vi "Basic Averaged DC-RMS for 1 Chan.vi"(7 "reset":bool, 8 "error in (no error)":errorcluster, 9 "window":T1(ring), 10 "averaging type":enum16{"Linear", "Exponential"}(ring), 11 "signal in":waveform(dbl)) -> (0 "error out":errorcluster, 2 "RMS value":dbl format="%0.2p", 3 "DC value":dbl format="%0.2p", 4 "measurement info":T2={"uncertainty"=0.0, "Warning"=FALSE, "comments"="reserved for future use"} {"uncertainty" format="%0.2p"})   [LabVIEW 2020, in "NI_MAPro.lvlib"]
doc: "Calculates the DC and RMS values of an input waveform or array of waveforms. This VI is similar to the Averaged DC-RMS VI, but this VI returns only one <B>DC value</B> and one <B>RMS value</B> per input waveform."
uses:
  NI_MAPro.lvlib
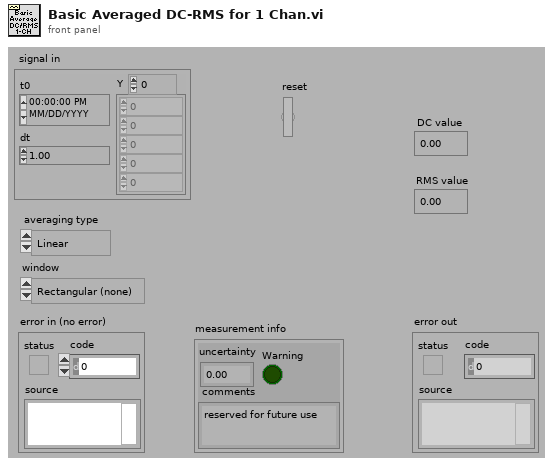
[diagram p1: front panel]
types:
  T1 = enum16{"Rectangular (none)", "Hanning", "Low side lobe"}
  T2 = cluster{"uncertainty":dbl, "Warning":bool, "comments":string}
  T3 = cluster{"DC history":dbl, "RMS history":dbl, "exp TC (samples)":dbl, "buffer size":i32, "t0 history":timestamp, "dt history":dbl, "timestamp":timestamp, "buffer":dbl[]}
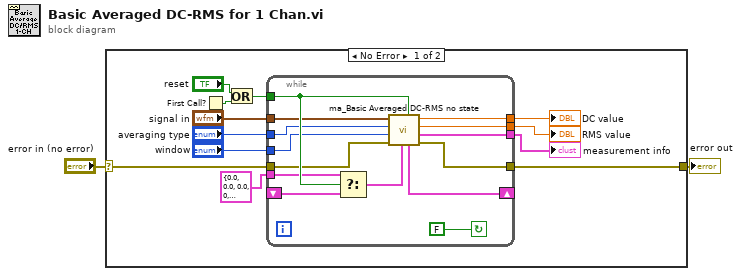
[diagram p0: block diagram]
diagram:
  n1 = case shown="No Error" "error in (no error)" {
    selector: "error in (no error)" -> [w3 w29]
    tunnel: [w8 w29] -> w2
    frame No Error {
      n2 = First Call?() -> (First Call?: T/F=w11:bool)
      n3 = Or(x="reset", y=w11) -> (x .or. y?=w9:bool)
      n4 = while {
        tunnel: T3 {"DC history"=0.0, "RMS history"=0.0, "exp TC (samples)"=0.0, "buffer size"=0, "t0 history"=timestamp(0 s since 1904-01-01), "dt history"=0.0, "timestamp"=timestamp(0 s since 1904-01-01), "buffer"=[]} ("state info") -> [w15]
        tunnel: [w19] -> w5
        tunnel: [w20] -> w6
        tunnel: [w21] -> w7
        tunnel: [w22] -> w8
        tunnel: w3 -> [w23]
        tunnel: w9 -> [w28]
        shift-left: _ -> [w16]
        shift-right: [w24] -> _
        tunnel: "window" -> [w25]
        tunnel: "averaging type" -> [w26]
        tunnel: "signal in" -> [w27]
        stop <- FALSE continue-if-true
        n5 = Select(t=w15, s=w28, f=w16) -> (s? t:f=w17:T3)
        n6 = call "ma_Basic Averaged DC-RMS no state.vi"("reset"=w28, "state info"=w17, "error in"=w23, "window"=w25, "averaging type"=w26, "signal in"=w27) -> ("error out"=w22:errorcluster, "measurement info cluster"=w21:T2, "RMS value"=w19:dbl, "DC value"=w20:dbl, "state info"=w24:T3)  [unwired: 1 in]
      }
      "DC value" <- w6
      "RMS value" <- w5
      "measurement info" <- w7
    }
    frame Error {
    }
  }
  "error out" <- w2
